vi "I2C_Decode_data.vi"(8 "Add points":dbl=10.0, 9 "VDDA 3":dbl=2.5, 10 "waveform":waveform(dbl), 11 "Index":dbl[](array[numeric])) -> (1 "Data Binary":bool[](array[boolean])=[TRUE, TRUE, TRUE, TRUE, TRUE, FALSE, FALSE, TRUE, TRUE, TRUE, FALSE, TRUE], 2 "Data ACK":bool, 3 "Data":u32=2975 format="%.0x")   [LabVIEW 2019]
panel:
  out "Array 4":dbl[](array[numeric])=[0.03750000000000009, 2.4360937499999995, 0.05249999999999977, -0.05343750000000025, -0.017343750000000213, 2.4328125, 0.20250000000000012, 0.06046875000000007, -0.07593750000000021, 2.4351562499999995, 0.1846874999999999, -0.005156250000000195, 0.0885937499999998, -0.0070312500000002665, 0.5826562500000003, 2.338125, 2.4604687499999995, 0.04921875000000009, 0.05484374999999986, 0.03374999999999995, -0.01171875, 2.3404687499999994, 0.46734374999999995, 0.03937500000000016, 0.06796874999999991, 0.06000000000000005, 0.012187500000000018, 2.40046875, 0.1471874999999998, 0.029999999999999805, 0.03234374999999989, 0.00749999999999984, 0.7846874999999995, 2.4553125, -0.053906250000000266, 0.012187500000000018, -0.07828124999999986, 2.3390625, -0.014531250000000107, -0.08765625000000021, 0.03374999999999995, -0.030468750000000266, 0.08390625000000007, 2.44125, 0.1143749999999999, 0.039843749999999734, -0.020624999999999893, 0.04078124999999977, 0.06421874999999977, 0.07499999999999973, 0.6703124999999996, 2.3864062500000003, 2.32125, 2.39953125]
  out "size(s) 3":i32=14
  out "subarray 2":dbl[](array[numeric])=[1.0, 0.0, 1.0, 1.0, 1.0, 0.0, 0.0, 1.0, 1.0, 1.0, 1.0, 1.0, 1.0, 1.0]
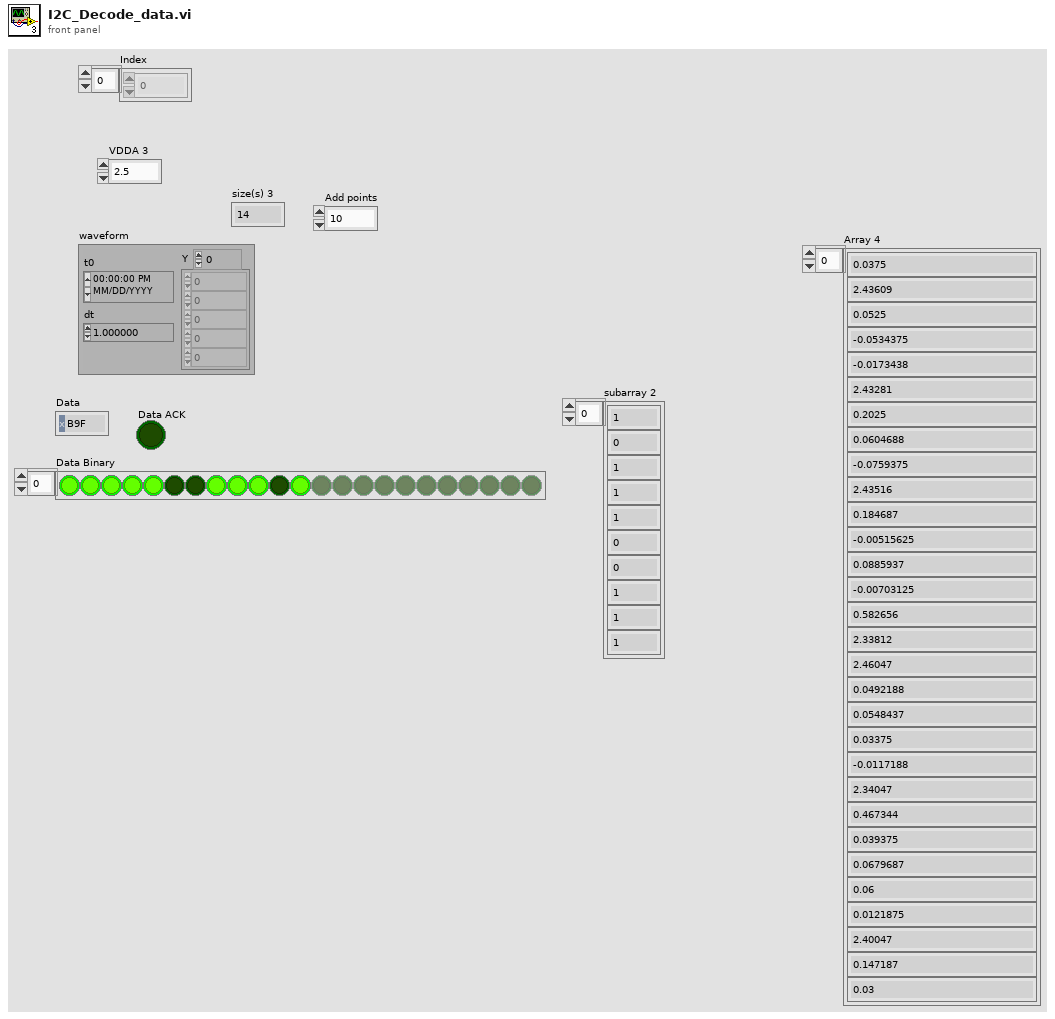
[diagram p1: front panel]
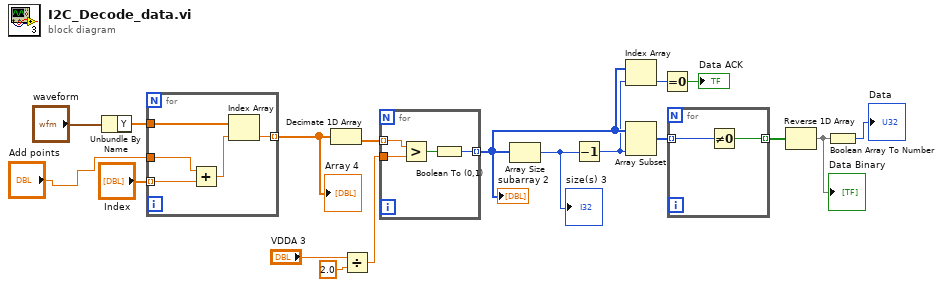
[diagram p0: block diagram]
diagram:
  n1 = Unbundle By Name("waveform") -> ("Y"=w5:dbl[])
  n2 = for {
    tunnel: "Index" -> [w22] mode=indexing
    tunnel: w5 -> [w23]
    tunnel: [w21] -> w18 mode=indexing
    tunnel: "Add points" -> [w19]
    n3 = Add(x=w19, y=w22) -> (x+y=w20:dbl)
    n4 = Index Array(array=w23, index=w20) -> (element=w21:dbl)
  }
  "Array 4" <- w18
  n5 = Decimate 1D Array(w18) -> (w17:dbl[])  [unwired: 1 out]
  n6 = Divide(x="VDDA 3", y=2.0) -> (x/y=w15:dbl)
  n7 = for {
    tunnel: w17 -> [w27] mode=indexing
    tunnel: w15 -> [w26]
    tunnel: [w24] -> w6 mode=indexing
    n8 = Greater?(x=w27, y=w26) -> (0:w25:bool)
    n9 = Boolean To (0,1)(Boolean=w25) -> (0, 1=w24:i16)
  }
  "subarray 2" <- w6
  n10 = Array Size(array=w6) -> (size(s)=w10:i32)
  "size(s) 3" <- w10
  n11 = Decrement(x=w10) -> (x-1=w4:i32)
  n12 = Index Array(array=w6, index=w4) -> (element=w11:i16)
  n13 = Array Subset(array=w6, length=w4) -> (w13:i16[])  [unwired: 1 in]
  n14 = Equal To 0?(x=w11) -> (x = 0?=→"Data ACK":bool)
  n15 = for {
    tunnel: w13 -> [w29] mode=indexing
    tunnel: [w28] -> w8 mode=indexing
    n16 = Not Equal To 0?(x=w29) -> (x != 0?=w28:bool)
  }
  n17 = Reverse 1D Array(array=w8) -> (reversed array=w7:bool[])
  "Data Binary" <- w7
  n18 = Boolean Array To Number(Boolean array=w7) -> (number=→"Data":u32)
